vi "debugging_Create.vi"(0 "reference in":refnum<class "debugging.lvclass">, 5 "error in (no error)":errorcluster) -> (14 "reference out":refnum<class "debugging.lvclass">, 19 "error out":errorcluster)   [LabVIEW 2019, in "debugging.lvclass"]
uses:
  debugging.lvclass
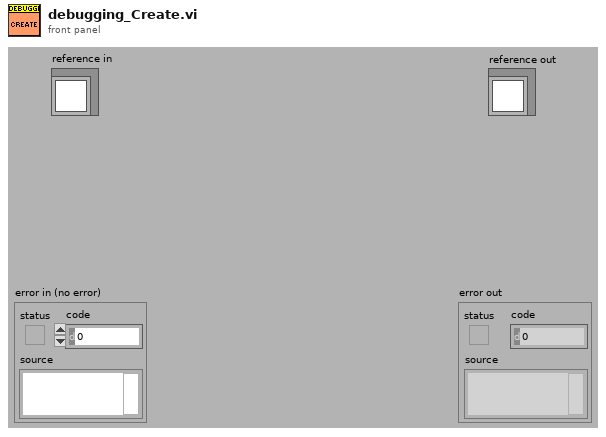
[diagram p1: front panel]
types:
  T1 = typedef "G4BaseTemplate_Simple_4x4x4.lvclass/ObjectAttributes.ctl" = cluster{"Attribute1":dbl}
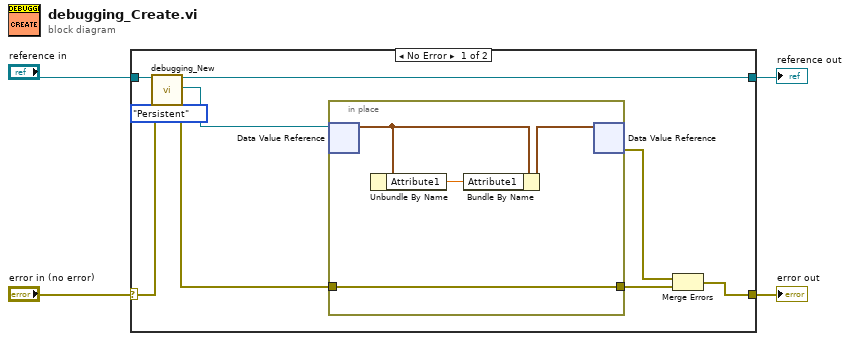
[diagram p0: block diagram]
diagram:
  n1 = case shown="No Error" "error in (no error)" {
    selector: "error in (no error)" -> [w12 w19]
    tunnel: [w9 w19] -> w3
    tunnel: "reference in" -> [w13 w18]
    tunnel: [w11 w18] -> w1
    frame No Error {
      n2 = call "debugging_New.vi"("reference in"=w13, "error in (no error)"=w12, "Persistent/Debugging(Default)"=enum16{"Default", "Persistent", "NonPersistent"}."Persistent") -> ("reference out"=w11:refnum<class "debugging.lvclass">, "DVRRefOut"=w8:refnum<data-value>, "error out"=w7:errorcluster)  [unwired: 13 in, 1 out]
      n3 = in-place {
        in-place-border: w7 -> [w14]
        in-place-border: [w14] -> w6
        n4 = in-place-dvr #1(w8) -> (w16:T1)  [unwired: 1 out]
        n5 = Unbundle By Name(w16) -> ("Attribute1"=w15:dbl)
        n6 = Bundle By Name(cluster=w16, "Attribute1"=w15) -> (w17:T1)
        n7 = in-place-dvr #1(w17) -> (w10:errorcluster)  [unwired: 1 out]
      }
      n8 = Merge Errors(w10, w6) -> (w9:errorcluster)
    }
    frame Error {
    }
  }
  "error out" <- w3
  "reference out" <- w1
